vi "finishKickoffEnemyPlayVSS.vi"(8 "error in (no error)":errorcluster, 10 "Game in":refnum<class "Game.lvclass">, 11 "KickoffEnemyPlayVSS in":refnum<class "KickoffEnemyPlayVSS.lvclass">) -> (0 "error out":errorcluster, 2 "result":bool, 3 "KickoffEnemyPlayVSS out":refnum<class "KickoffEnemyPlayVSS.lvclass">)   [LabVIEW 2020, in "KickoffEnemyPlayVSS.lvclass"]
uses:
  KickoffEnemyPlayVSS.lvclass
  Game_class/Game.lvclass
  Game_class/Game.lvclass/Game.ctl
  Events_class/Events.lvclass/Events.ctl
  Game_class/Read Referee.vi
  Game_class/Read EventsRef.vi
  Events_class/Read touch.vi
  Referee_class/Referee.lvclass
  Events_class/Events.lvclass
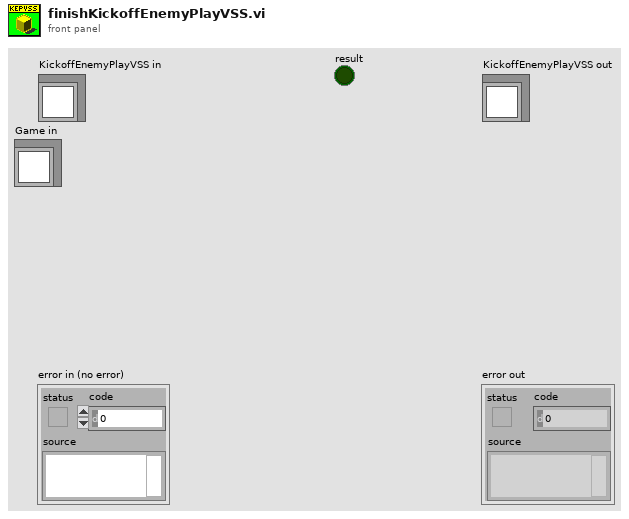
[diagram p1: front panel]
types:
  T1 = enum16{"AUTO", "GAME_ON", "STOP", "KICKOFF", "FREE_BALL", "GOAL_KICK", "PENALTY_KICK", "FREE_KICK"}
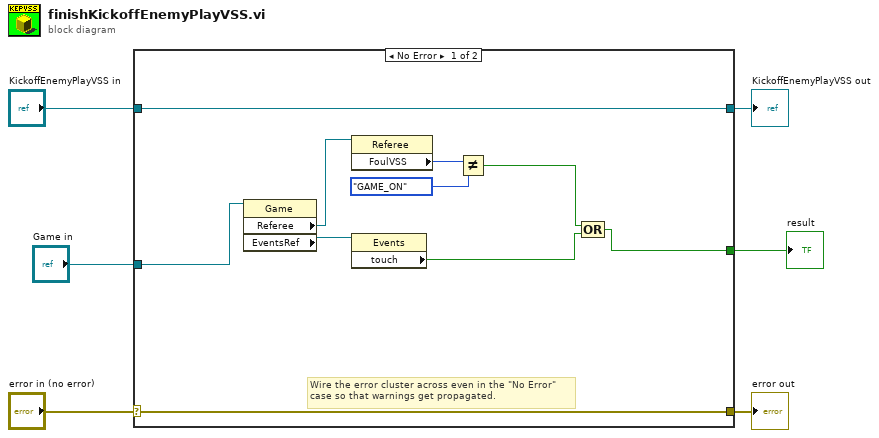
[diagram p0: block diagram]
diagram:
  n1 = case shown="No Error" "error in (no error)" {
    selector: "error in (no error)" -> [w15 w18]
    tunnel: [w15 w18] -> w5
    tunnel: [w16 w17] -> w3
    tunnel: "KickoffEnemyPlayVSS in" -> [w16 w17]
    tunnel: "Game in" -> [w14 _]
    tunnel: [w12 _] -> w1
    frame No Error {
      # "Wire the error cluster across even in the \"No Error\"\ncase so that warnings get propagated."
      n2 = property class="Game"(reference=w14) -> ("Referee"=w9:refnum<class "Referee.lvclass">, "EventsRef"=w13:refnum<class "Events.lvclass">)  [unwired: 1 in, 2 out]
      n3 = property class="Referee"(reference=w9) -> ("FoulVSS"=w11:T1)  [unwired: 1 in, 2 out]
      n4 = property class="Events"(reference=w13) -> ("touch"=w7:bool)  [unwired: 1 in, 2 out]
      n5 = Not Equal?(x=w11, y=T1."GAME_ON") -> (x != y?=w8:bool)
      n6 = Compound Arithmetic op=OR(w8, w7) -> (w12:bool)
    }
    frame Error {
    }
  }
  "error out" <- w5
  "KickoffEnemyPlayVSS out" <- w3
  "result" <- w1
